vi "Differentiation (1 Ch).vi"(8 "error in (no error)":errorcluster, 10 "differentiation type":T1(ring)=enum."single differentiation", 11 "Signal":waveform(sgl)) -> (0 "error out":errorcluster, 2 "Differentiated Signal":waveform(sgl))   [LabVIEW 2017, in "VibrationAnalysisFunctions.lvlib"]
uses:
  <vilib>/addons/InsightCM/Utilities/Analysis/Vibration/VibrationAnalysisFunctions.lvlib
  <vilib>/ptbypt/NI_PtbyPt.lvlib
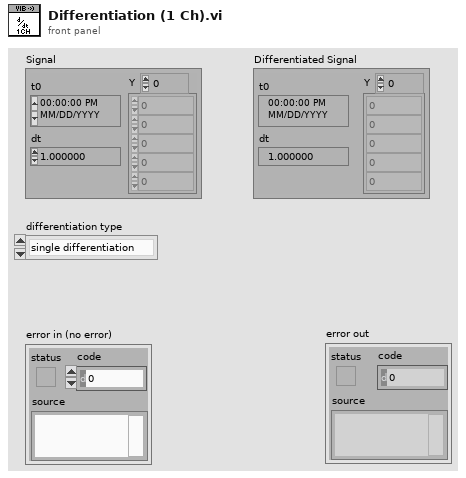
[diagram p1: front panel]
types:
  T1 = enum16{"single integration", "double integration", "single differentiation", "double differentiation", "none"}
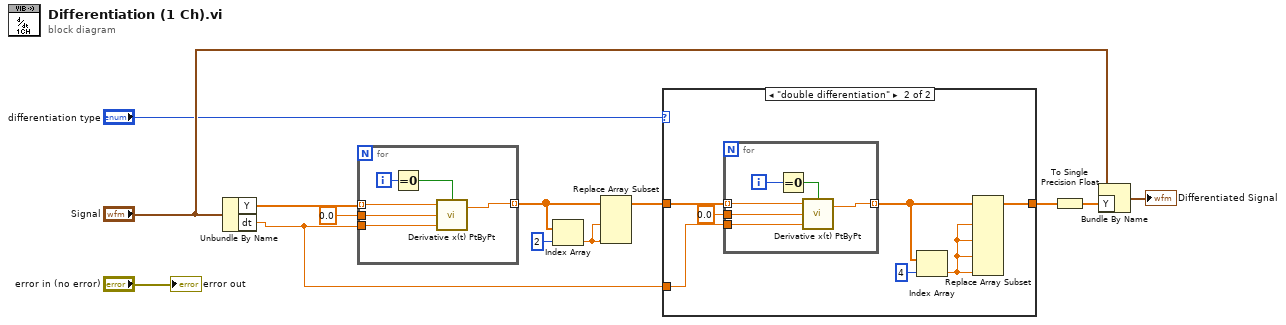
[diagram p0: block diagram]
diagram:
  n1 = Unbundle By Name("Signal") -> ("Y"=w6:sgl[], "dt"=w3:dbl)
  n2 = for {
    tunnel: w6 -> [w19] mode=indexing
    tunnel: w3 -> [w18]
    tunnel: [w17] -> w12 mode=indexing
    tunnel: 0.0 -> [w16]
    i -> [w15]
    n3 = Equal To 0?(x=w15) -> (x = 0?=w14:bool)
    n4 = call <vilib>:"Derivative x(t) PtByPt.vi"("initialize"=w14, "dt"=w18, "initial condition"=w16, "x"=w19) -> ("dx/dt"=w17:dbl)  [unwired: 1 out]
  }
  n5 = Index Array(array=w12, index=2) -> (element=w5:dbl)
  n6 = Replace Array Subset(array=w12, new element #1=w5, new element #2=w5) -> (w9:dbl[])  [unwired: 2 in]
  n7 = case shown="\"double differentiation\"" "differentiation type" {
    tunnel: w9 -> [w20 w27]
    tunnel: w3 -> [_ w26]
    tunnel: [w20 w23] -> w2
    frame "single differentiation", Default {
    }
    frame "double differentiation" {
      n8 = for {
        tunnel: w27 -> [w31] mode=indexing
        tunnel: w26 -> [w30]
        tunnel: [w29] -> w24 mode=indexing
        tunnel: 0.0 ("dx/dt") -> [w28]
        i -> [w32]
        n9 = Equal To 0?(x=w32) -> (x = 0?=w33:bool)
        n10 = call <vilib>:"Derivative x(t) PtByPt.vi"("initialize"=w33, "dt"=w30, "initial condition"=w28, "x"=w31) -> ("dx/dt"=w29:dbl)  [unwired: 1 out]
      }
      n11 = Index Array(array=w24, index=4) -> (element=w22:dbl)
      n12 = Replace Array Subset(array=w24, new element #1=w22, new element #2=w22, new element #3=w22, new element #4=w22) -> (w23:dbl[])  [unwired: 4 in]
    }
  }
  n13 = To Single Precision Float(number=w2) -> (single precision float=w1:sgl[])
  n14 = Bundle By Name(cluster="Signal", "Y"=w1) -> (→"Differentiated Signal":waveform(sgl))
  "error out" <- "error in (no error)"
